vi "Begin.vi"(8 "error in":errorcluster) -> (0 "error out":errorcluster)   [LabVIEW 2020]
doc: "Called before other user functions, this VI is expected to open initial I/O refnums, load in file data, and do all program initialization. Notice that the <B>error out</B> terminal is simply used for data flow. Wiring it to other structures or subVIs ensures that this VI runs first."
uses:
  <vilib>/Rock Robotics/WPI/DriverStation/WPI_DriverStationRobotMode2.ctl
  <vilib>/Rock Robotics/WPI/Joystick/WPI_JoystickDeviceEnum.ctl
  <vilib>/Rock Robotics/WPI/RobotDrive/WPI_RobotDriveDevRef.ctl
  <vilib>/Rock Robotics/WPI/MotorControl/WPI_MotorControlDeviceRef.ctl
  <vilib>/Rock Robotics/WPI/MotorControl/WPI_MotorControlType.ctl
  <vilib>/Rock Robotics/SystemInterfaces/DIO/FPGA_DIOPWMChannel.ctl
  <vilib>/Rock Robotics/WPI/PWM/WPI_PWMDeadband.ctl
  <vilib>/Rock Robotics/SystemInterfaces/DIO/FPGA_DIOChannel.ctl
  <vilib>/Rock Robotics/WPI/SafetyOutput/WPI_SafetyOutputConfigMenu.ctl
  <vilib>/Rock Robotics/WPI/ThirdParty/Phoenix-LabVIEW/Motor Controller/Controls/CTRE_Phoenix_MotorControl_FeedbackDevice.ctl
  <vilib>/Rock Robotics/WPI/ThirdParty/Phoenix-LabVIEW/Motor Controller/Controls/CTRE_Phoenix_MotorControl_NeutralMode.ctl
  <vilib>/Rock Robotics/SystemInterfaces/AI/FPGA_AIChannel.ctl
  <vilib>/Rock Robotics/WPI/ThirdParty/REV Robotics/REVLib/Typedef/Spark MAX Idle Mode.ctl
  Robot Global Data.vi
  <vilib>/Rock Robotics/Network Tables/NT Write String Array.vi
  <vilib>/Rock Robotics/WPI/Switch/WPI_SwitchOpenLimit.vi
  <vilib>/Rock Robotics/WPI/RobotDrive/WPI_RobotDriveOpen2MotorWithTalonSRX.vi
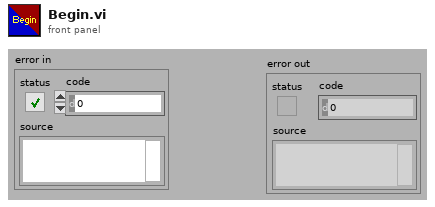
[diagram p1: front panel]
types:
  T1 = typedef "Spark MAX Idle Mode.ctl" = enum16{"Coast", "Brake"}
  T2 = typedef "FPGA_DIOChannel.ctl" = enum8{"DIO 0", "DIO 1", "DIO 2", "DIO 3", "DIO 4", "DIO 5", "DIO 6", "DIO 7", "DIO 8", "DIO 9", "DIO MXP 0", "DIO MXP 1", "DIO MXP 2", "DIO MXP 3", "DIO MXP 4", "DIO MXP 5", "DIO MXP 6", "DIO MXP 7", "DIO MXP 8", "DIO MXP 9", "DIO MXP 10", "DIO MXP 11", "DIO MXP 12", "DIO MXP 13", "DIO MXP 14", "DIO MXP 15", "SPI Port CS1", "SPI Port CS2", "SPI Port CS3", "SPI Port MISO", "SPI Port MOSI", "Invalid"}
  T3 = typedef "FPGA_AIChannel.ctl" = enum8{"AI 0", "AI 1", "AI 2", "AI 3", "AI MXP 0", "AI MXP 1", "AI MXP 2", "AI MXP 3", "Invalid"}
  T4 = typedef "CTRE_Phoenix_MotorControl_FeedbackDevice.ctl" = i8
  T5 = typedef "CTRE_Phoenix_MotorControl_NeutralMode.ctl" = enum8{"EEPROMSetting", "Override to Coast", "Override to Brake"}
  T6 = typedef "WPI_SafetyOutputConfigMenu.ctl" = enum16{"Enable", "Disable"}
  T7 = typedef "WPI_RobotDriveDevRef.ctl" = cluster{"DevStatus":errorcluster, "Motors[]":T8[], "Square Inputs":bool, "Max Output":dbl}
  T8 = typedef "WPI_MotorControlDeviceRef.ctl" = cluster{"DeviceStatus":errorcluster, "Type":T9, "PWM":cluster{"PWM Channel":T10, "DeadBand":T11}, "CAN":cluster{"Device Number":u8, "SetOutput VI Ref":variant, "GetOutput VI Ref":variant, "Enable VI Ref":variant, "Disable VI Ref":variant, "Data":variant}, "Invert":bool, "DIO PWM":cluster{"PWM \"Enable\" Channel":T10, "DIOChannel":T2, "PWM Rate":dbl}}
  T9 = typedef "WPI_MotorControlType.ctl" = enum16{"PWM", "CAN", "DIO PWM"}
  T10 = typedef "FPGA_DIOPWMChannel.ctl" = enum8{"PWM 0", "PWM 1", "PWM 2", "PWM 3", "PWM 4", "PWM 5", "PWM 6", "PWM 7", "PWM 8", "PWM 9", "PWM MXP 0", "PWM MXP 1", "PWM MXP 2", "PWM MXP 3", "PWM MXP 4", "PWM MXP 5", "PWM MXP 6", "PWM MXP 7", "PWM MXP 8", "PWM MXP 9", "Invalid"}
  T11 = typedef "WPI_PWMDeadband.ctl" = cluster{"Name":string, "maxPositivePwm":i32, "minPositivePwm":i32, "centerPwm":i32, "maxNegativePwm":i32, "minNegativePwm":i32, "angularRange":u16}
  T12 = typedef "WPI_JoystickDeviceEnum.ctl" = enum16{"USB 0", "USB 1", "USB 2", "USB 3", "USB 4", "USB 5"}
  T13 = typedef "WPI_DriverStationRobotMode2.ctl" = enum16{"Autonomous Disabled", "Autonomous Enabled", "Teleop Disabled", "Teleop Enabled", "Disconnected", "Finish", "Test Disabled", "Test Enabled", "Emergency Stopped"}
  T14 = typedef "WPI_SwitchDevRef.ctl" = cluster{"DevStatus":errorcluster, "DIO Channel":T2, "CntIndex":T15, "Normally Closed":bool}
  T15 = typedef "FPGA_CounterCtrSystemIndex.ctl" = enum8{"Ctr 0", "Ctr 1", "Ctr 2", "Ctr 3", "Ctr 4", "Ctr 5", "Ctr 6", "Ctr 7", "Invalid"}
  T16 = typedef "WPI_JoystickDevRef.ctl" = cluster{"Device":T12}
  T17 = typedef "WPI_AnalogChannelDevRef.ctl" = cluster{"DevStatus":errorcluster, "Analog Channel":T3}
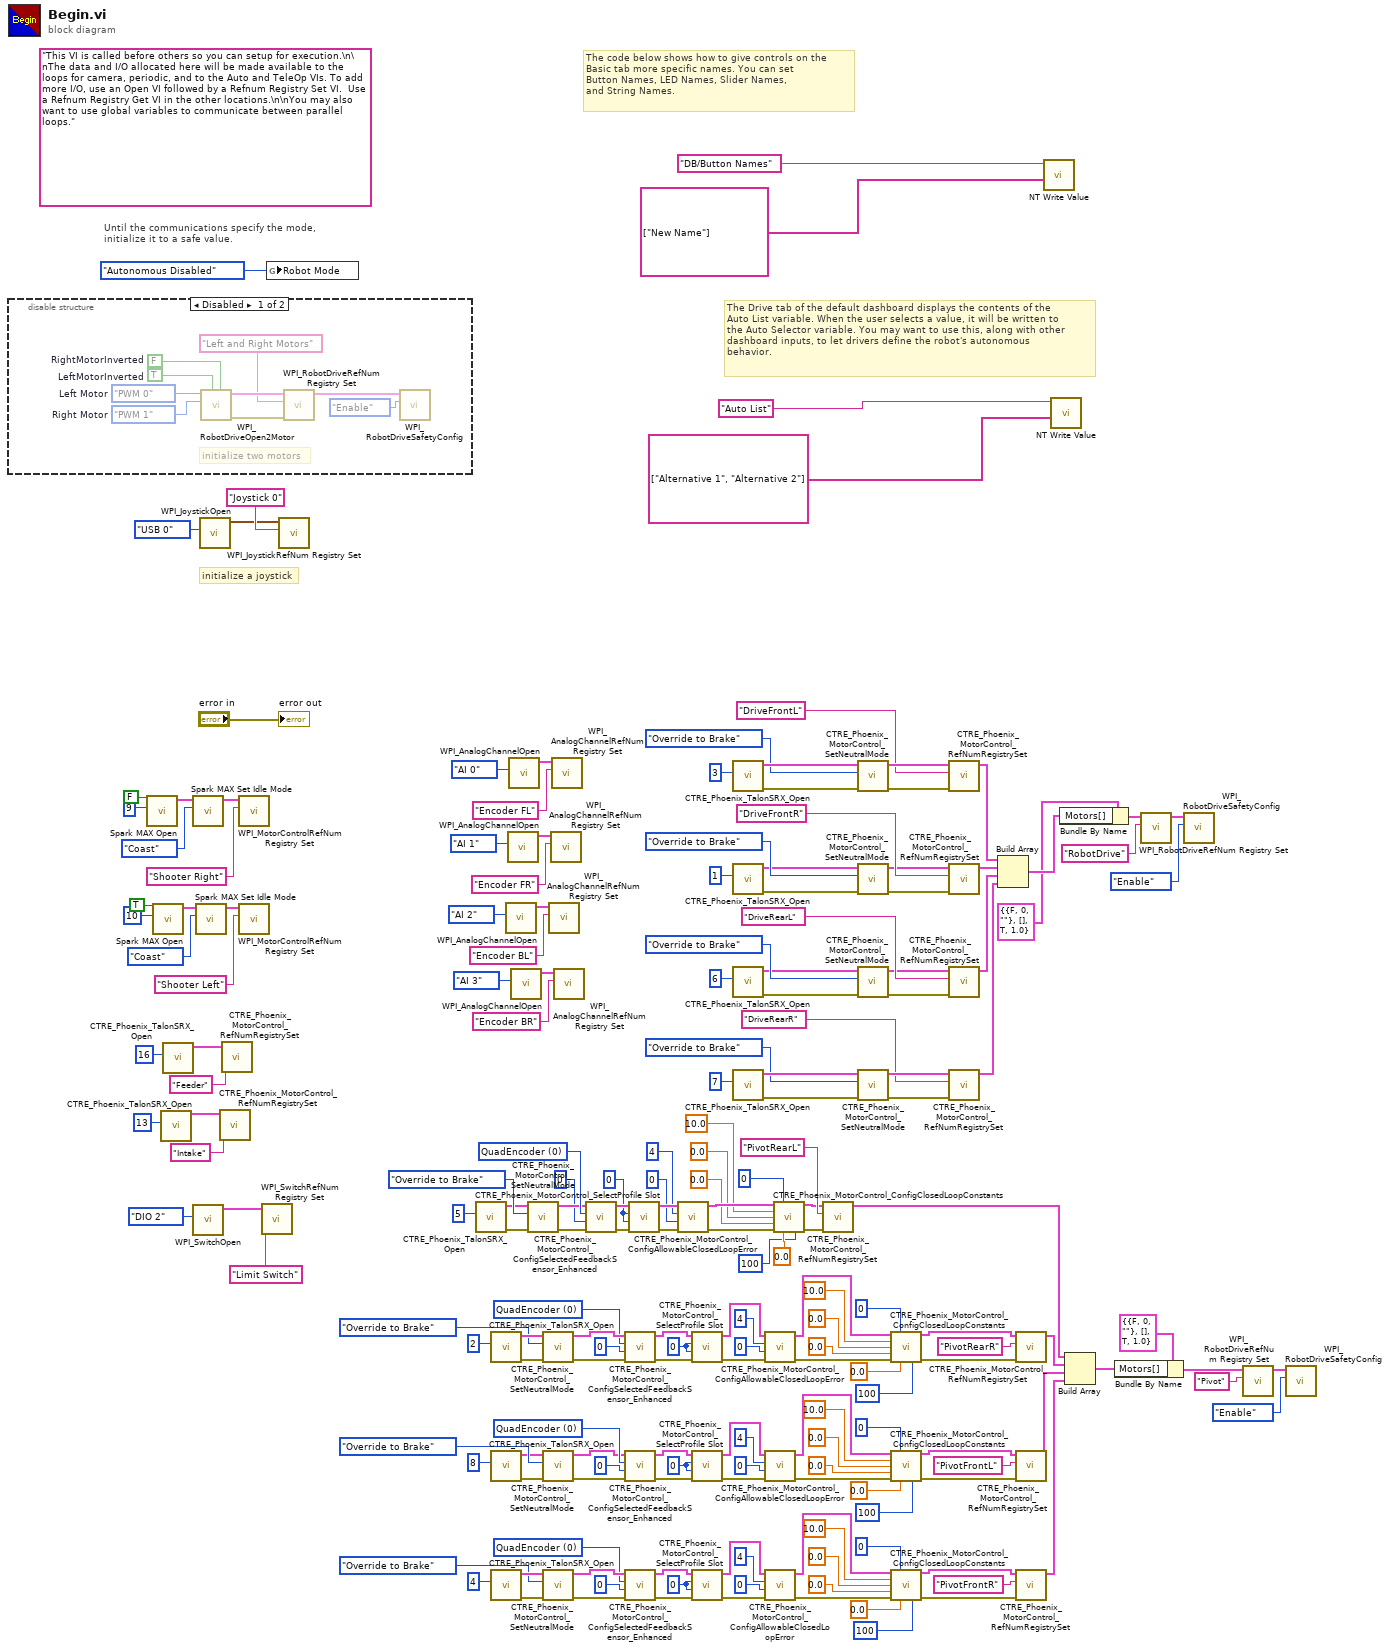
[diagram p0: block diagram]
diagram:
  w50 = 0 ("slotIdx")
  w43 = T4 0 items=["QuadEncoder"=0, "Analog"=2, "Tachometer"=4, "Pulse Width Encoded Position"=8, "Sensor Sum (S0 + S1)"=9, "Sensor Difference (D0 - D1)"=10, "Remote Source 0"=11, "Remote Source 1"=12, "Software Emulated"=15] ("Feedback Device")
  w75 = 0 ("slotIdx")
  w82 = T4 0 items=["QuadEncoder"=0, "Analog"=2, "Tachometer"=4, "Pulse Width Encoded Position"=8, "Sensor Sum (S0 + S1)"=9, "Sensor Difference (D0 - D1)"=10, "Remote Source 0"=11, "Remote Source 1"=12, "Software Emulated"=15] ("Feedback Device")
  w96 = 0 ("slotIdx")
  w89 = T4 0 items=["QuadEncoder"=0, "Analog"=2, "Tachometer"=4, "Pulse Width Encoded Position"=8, "Sensor Sum (S0 + S1)"=9, "Sensor Difference (D0 - D1)"=10, "Remote Source 0"=11, "Remote Source 1"=12, "Software Emulated"=15] ("Feedback Device")
  w123 = 0 ("slotIdx")
  w130 = T4 0 items=["QuadEncoder"=0, "Analog"=2, "Tachometer"=4, "Pulse Width Encoded Position"=8, "Sensor Sum (S0 + S1)"=9, "Sensor Difference (D0 - D1)"=10, "Remote Source 0"=11, "Remote Source 1"=12, "Software Emulated"=15] ("Feedback Device")
  (unwired) "This VI is called before others so you can setup for execution.\n\nThe data and I/O allocated here will be made available to the loops for camera, periodic, and to the Auto and TeleOp VIs. To add more I/O, use an Open VI followed by a Refnum Registry Set VI.  Use a Refnum Registry Get VI in the other locations.\n\nYou may also want to use global variables to communicate between parallel loops."
  # "The Drive tab of the default dashboard displays the contents of the\nAuto List variable. When the user selects a value, it will be written to\nthe Auto Selector variable. You may want to use this, along with other\ndashboard inputs, to let drivers define the robot's autonomous\nbehavior."
  # "The code below shows how to give controls on the\nBasic tab more specific names. You can set\nButton Names, LED Names, Slider Names,\nand String Names."
  # "initialize a joystick"
  # "Until the communications specify the mode,\ninitialize it to a safe value."
  n1 = disable-structure shown="Disabled" {
    frame Disabled {
      w197 = FPGA_DIOPWMChannel."PWM 1"  # Right Motor
      w198 = FPGA_DIOPWMChannel."PWM 0"  # Left Motor
      w202 = TRUE  # LeftMotorInverted
      w203 = FALSE  # RightMotorInverted
      # "initialize two motors"
      n2 = call-poly <vilib>:"WPI_RobotDriveOpen2Motor.vi"("Right Motor Inverted"=w203, "Left Motor Inverted"=w202, "Right Motor"=w197, "Left Motor"=w198) -> ("error out"=w199:errorcluster, "RobotDriveDevRef"=w201:T7)  [unwired: 1 in, 5 out]
      n3 = call <vilib>:"WPI_RobotDriveRefNum Registry Set.vi"("error in (no error)"=w199, "refnum name"="Left and Right Motors", "RobotDriveDevRef"=w201) -> ("RobotDriveDevRef"=w196:T7)  [unwired: 1 in, 7 out]
      n4 = call <vilib>:"WPI_RobotDriveSafetyConfig.vi"("mode"=WPI_SafetyOutputConfigMenu."Enable", "RobotDriveDevRef"=w196) -> ()  [unwired: 8 in, 2 out]
    }
    frame Enabled {
    }
  }
  n5 = call <vilib>:"Spark MAX Open.vi"("Invert"=FALSE, "Device Number"=u8 9) -> ("MotorControlDeviceRef"=w7:T8)  [unwired: 8 in, 1 out]
  n6 = call <vilib>:"Spark MAX Open.vi"("Invert"=TRUE, "Device Number"=u8 10) -> ("MotorControlDeviceRef"=w5:T8)  [unwired: 8 in, 1 out]
  n7 = call <vilib>:"CTRE_Phoenix_TalonSRX_Open.vi"("Device Number"=u8 13) -> ("PhoenixMotorControlDevRef"=w9:T8)  [unwired: 9 in, 1 out]
  n8 = call <vilib>:"CTRE_Phoenix_TalonSRX_Open.vi"("Device Number"=u8 16) -> ("PhoenixMotorControlDevRef"=w16:T8)  [unwired: 9 in, 1 out]
  n9 = call <vilib>:"Spark MAX Set Idle Mode.vi"("Idle Mode"=Spark_MAX_Idle_Mode."Coast", "MotorControlDeviceRef in"=w7) -> ("MotorControlDeviceRef out"=w6:T8)  [unwired: 8 in, 1 out]
  n10 = call-poly <vilib>:"WPI_SwitchOpen.vi"("DIO Channel"=FPGA_DIOChannel."DIO 2") -> ("SwitchDevRef"=w11:T14)  [unwired: 9 in, 1 out]
  n11 = call <vilib>:"Spark MAX Set Idle Mode.vi"("Idle Mode"=Spark_MAX_Idle_Mode."Coast", "MotorControlDeviceRef in"=w5) -> ("MotorControlDeviceRef out"=w3:T8)  [unwired: 8 in, 1 out]
  n12 = call <vilib>:"WPI_JoystickOpen.vi"("JoystickDevice"=WPI_JoystickDeviceEnum."USB 0") -> ("JoystickDevRef"=w192:T16)  [unwired: 10 in]
  n13 = call <vilib>:"CTRE_Phoenix_MotorControl_RefNumRegistrySet.vi"("refnum name"="Intake", "PhoenixMotorControlDevRef"=w9) -> ()  [unwired: 8 in, 2 out]
  n14 = call <vilib>:"CTRE_Phoenix_MotorControl_RefNumRegistrySet.vi"("refnum name"="Feeder", "PhoenixMotorControlDevRef"=w16) -> ()  [unwired: 8 in, 2 out]
  n15 = call <vilib>:"WPI_MotorControlRefNum Registry Set.vi"("refnum name"="Shooter Right", "MotorControlDevRef"=w6) -> ()  [unwired: 8 in, 2 out]
  n16 = call <vilib>:"WPI_MotorControlRefNum Registry Set.vi"("refnum name"="Shooter Left", "MotorControlDevRef"=w3) -> ()  [unwired: 8 in, 2 out]
  n17 = call <vilib>:"WPI_SwitchRefNum Registry Set.vi"("refnum name"="Limit Switch", "SwitchDevRef"=w11) -> ()  [unwired: 8 in, 2 out]
  n18 = global write "Robot Global Data.vi" "Robot Mode"(WPI_DriverStationRobotMode2."Autonomous Disabled" ("Robot Mode")) -> ()
  n19 = call <vilib>:"WPI_JoystickRefNum Registry Set.vi"("refnum name"="Joystick 0", "JoystickDevRef"=w192) -> ()  [unwired: 8 in, 2 out]
  n20 = call <vilib>:"CTRE_Phoenix_TalonSRX_Open.vi"("Device Number"=5) -> ("error out"=w127:errorcluster, "PhoenixMotorControlDevRef"=w164:T8)  [unwired: 9 in]
  n21 = call <vilib>:"CTRE_Phoenix_TalonSRX_Open.vi"("Device Number"=2) -> ("error out"=w92:errorcluster, "PhoenixMotorControlDevRef"=w87:T8)  [unwired: 9 in]
  n22 = call <vilib>:"CTRE_Phoenix_TalonSRX_Open.vi"("Device Number"=8) -> ("error out"=w79:errorcluster, "PhoenixMotorControlDevRef"=w84:T8)  [unwired: 9 in]
  n23 = call <vilib>:"CTRE_Phoenix_TalonSRX_Open.vi"("Device Number"=4) -> ("error out"=w46:errorcluster, "PhoenixMotorControlDevRef"=w41:T8)  [unwired: 9 in]
  n24 = call <vilib>:"WPI_AnalogChannelOpen.vi"("Analog Channel"=FPGA_AIChannel."AI 2") -> ("AIDeviceRef"=w28:T17)  [unwired: 9 in, 1 out]
  n25 = call <vilib>:"WPI_AnalogChannelOpen.vi"("Analog Channel"=FPGA_AIChannel."AI 1") -> ("AIDeviceRef"=w25:T17)  [unwired: 9 in, 1 out]
  n26 = call <vilib>:"WPI_AnalogChannelOpen.vi"("Analog Channel"=FPGA_AIChannel."AI 0") -> ("AIDeviceRef"=w23:T17)  [unwired: 9 in, 1 out]
  n27 = call <vilib>:"WPI_AnalogChannelOpen.vi"("Analog Channel"=FPGA_AIChannel."AI 3") -> ("AIDeviceRef"=w29:T17)  [unwired: 9 in, 1 out]
  n28 = call <vilib>:"CTRE_Phoenix_MotorControl_SetNeutralMode.vi"("error in (no error)"=w127, "Motor Control Neutral Mode"=CTRE_Phoenix_MotorControl_NeutralMode."Override to Brake", "PhoenixMotorControlDevRef"=w164) -> ("error out"=w126:errorcluster, "PhoenixMotorControlDevRef"=w129:T8)  [unwired: 7 in]
  n29 = call <vilib>:"CTRE_Phoenix_MotorControl_SetNeutralMode.vi"("error in (no error)"=w92, "Motor Control Neutral Mode"=CTRE_Phoenix_MotorControl_NeutralMode."Override to Brake", "PhoenixMotorControlDevRef"=w87) -> ("error out"=w93:errorcluster, "PhoenixMotorControlDevRef"=w90:T8)  [unwired: 7 in]
  n30 = call <vilib>:"CTRE_Phoenix_MotorControl_SetNeutralMode.vi"("error in (no error)"=w79, "Motor Control Neutral Mode"=CTRE_Phoenix_MotorControl_NeutralMode."Override to Brake", "PhoenixMotorControlDevRef"=w84) -> ("error out"=w78:errorcluster, "PhoenixMotorControlDevRef"=w81:T8)  [unwired: 7 in]
  n31 = call <vilib>:"CTRE_Phoenix_MotorControl_SetNeutralMode.vi"("error in (no error)"=w46, "Motor Control Neutral Mode"=CTRE_Phoenix_MotorControl_NeutralMode."Override to Brake", "PhoenixMotorControlDevRef"=w41) -> ("error out"=w47:errorcluster, "PhoenixMotorControlDevRef"=w44:T8)  [unwired: 7 in]
  n32 = call <vilib>:"WPI_AnalogChannelRefNum Registry Set.vi"("refnum name"="Encoder BL", "AIDeviceRef"=w28) -> ()  [unwired: 8 in, 2 out]
  n33 = call <vilib>:"WPI_AnalogChannelRefNum Registry Set.vi"("refnum name"="Encoder FR", "AIDeviceRef"=w25) -> ()  [unwired: 8 in, 2 out]
  n34 = call <vilib>:"WPI_AnalogChannelRefNum Registry Set.vi"("refnum name"="Encoder FL", "AIDeviceRef"=w23) -> ()  [unwired: 8 in, 2 out]
  n35 = call <vilib>:"WPI_AnalogChannelRefNum Registry Set.vi"("refnum name"="Encoder BR", "AIDeviceRef"=w29) -> ()  [unwired: 8 in, 2 out]
  n36 = call <vilib>:"CTRE_Phoenix_MotorControl_ConfigSelectedFeedbackSensor_Enhanced.vi"("error in (no error)"=w126, "pidLoopIdx"=0, "Feedback Device"=w130, "PhoenixMotorControlDevRef"=w129) -> ("error out"=w125:errorcluster, "PhoenixMotorControlDevRef"=w124:T8)  [unwired: 6 in]
  n37 = call <vilib>:"CTRE_Phoenix_MotorControl_ConfigSelectedFeedbackSensor_Enhanced.vi"("error in (no error)"=w93, "pidLoopIdx"=0, "Feedback Device"=w89, "PhoenixMotorControlDevRef"=w90) -> ("error out"=w94:errorcluster, "PhoenixMotorControlDevRef"=w95:T8)  [unwired: 6 in]
  n38 = call <vilib>:"CTRE_Phoenix_MotorControl_ConfigSelectedFeedbackSensor_Enhanced.vi"("error in (no error)"=w78, "pidLoopIdx"=0, "Feedback Device"=w82, "PhoenixMotorControlDevRef"=w81) -> ("error out"=w77:errorcluster, "PhoenixMotorControlDevRef"=w76:T8)  [unwired: 6 in]
  n39 = call <vilib>:"CTRE_Phoenix_MotorControl_ConfigSelectedFeedbackSensor_Enhanced.vi"("error in (no error)"=w47, "pidLoopIdx"=0, "Feedback Device"=w43, "PhoenixMotorControlDevRef"=w44) -> ("error out"=w48:errorcluster, "PhoenixMotorControlDevRef"=w49:T8)  [unwired: 6 in]
  n40 = call <vilib>:"CTRE_Phoenix_MotorControl_SelectProfile Slot.vi"("error in (no error)"=w125, "pidLoopIdx"=w123, "slotIdx"=w123, "PhoenixMotorControlDevRef"=w124) -> ("error out"=w122:errorcluster, "PhoenixMotorControlDevRef"=w121:T8)  [unwired: 6 in]
  n41 = call <vilib>:"CTRE_Phoenix_MotorControl_ConfigAllowableClosedLoopError.vi"("error in (no error)"=w122, "slotIdx"=u32 0, "allowableClosedLoopError"=4, "PhoenixMotorControlDevRef"=w121) -> ("error out"=w117:errorcluster, "PhoenixMotorControlDevRef"=w118:T8)  [unwired: 6 in]
  n42 = call <vilib>:"CTRE_Phoenix_MotorControl_SelectProfile Slot.vi"("error in (no error)"=w94, "pidLoopIdx"=w96, "slotIdx"=w96, "PhoenixMotorControlDevRef"=w95) -> ("error out"=w97:errorcluster, "PhoenixMotorControlDevRef"=w98:T8)  [unwired: 6 in]
  n43 = call <vilib>:"CTRE_Phoenix_MotorControl_SelectProfile Slot.vi"("error in (no error)"=w77, "pidLoopIdx"=w75, "slotIdx"=w75, "PhoenixMotorControlDevRef"=w76) -> ("error out"=w74:errorcluster, "PhoenixMotorControlDevRef"=w73:T8)  [unwired: 6 in]
  n44 = call <vilib>:"CTRE_Phoenix_MotorControl_SelectProfile Slot.vi"("error in (no error)"=w48, "pidLoopIdx"=w50, "slotIdx"=w50, "PhoenixMotorControlDevRef"=w49) -> ("error out"=w51:errorcluster, "PhoenixMotorControlDevRef"=w52:T8)  [unwired: 6 in]
  n45 = call <vilib>:"CTRE_Phoenix_TalonSRX_Open.vi"("Device Number"=3) -> ("error out"=w182:errorcluster, "PhoenixMotorControlDevRef"=w181:T8)  [unwired: 9 in]
  n46 = call <vilib>:"CTRE_Phoenix_TalonSRX_Open.vi"("Device Number"=1) -> ("error out"=w157:errorcluster, "PhoenixMotorControlDevRef"=w158:T8)  [unwired: 9 in]
  n47 = call <vilib>:"CTRE_Phoenix_TalonSRX_Open.vi"("Device Number"=6) -> ("error out"=w143:errorcluster, "PhoenixMotorControlDevRef"=w144:T8)  [unwired: 9 in]
  n48 = call <vilib>:"CTRE_Phoenix_TalonSRX_Open.vi"("Device Number"=7) -> ("error out"=w150:errorcluster, "PhoenixMotorControlDevRef"=w149:T8)  [unwired: 9 in]
  n49 = call <vilib>:"CTRE_Phoenix_MotorControl_ConfigAllowableClosedLoopError.vi"("error in (no error)"=w97, "slotIdx"=u32 0, "allowableClosedLoopError"=4, "PhoenixMotorControlDevRef"=w98) -> ("error out"=w102:errorcluster, "PhoenixMotorControlDevRef"=w101:T8)  [unwired: 6 in]
  n50 = call <vilib>:"CTRE_Phoenix_MotorControl_ConfigAllowableClosedLoopError.vi"("error in (no error)"=w74, "slotIdx"=u32 0, "allowableClosedLoopError"=4, "PhoenixMotorControlDevRef"=w73) -> ("error out"=w69:errorcluster, "PhoenixMotorControlDevRef"=w70:T8)  [unwired: 6 in]
  n51 = call <vilib>:"CTRE_Phoenix_MotorControl_ConfigAllowableClosedLoopError.vi"("error in (no error)"=w51, "slotIdx"=u32 0, "allowableClosedLoopError"=4, "PhoenixMotorControlDevRef"=w52) -> ("error out"=w56:errorcluster, "PhoenixMotorControlDevRef"=w55:T8)  [unwired: 6 in]
  n52 = call <vilib>:"CTRE_Phoenix_MotorControl_ConfigClosedLoopConstants.vi"("PhoenixMotorControlDevRef"=w118, "slotIdx"=0, "P"=10.0, "I"=0.0, "D"=0.0, "error in (no error)"=w117, "F"=0.0, "timeoutMs"=100) -> ("PhoenixMotorControlDevRef"=w110:T8, "error out"=w109:errorcluster)  [unwired: 6 in]
  n53 = call <vilib>:"CTRE_Phoenix_MotorControl_RefNumRegistrySet.vi"("error in (no error)"=w109, "refnum name"="PivotRearL", "PhoenixMotorControlDevRef"=w110) -> ("PhoenixMotorControlDevRef"=w170:T8)  [unwired: 7 in, 1 out]
  n54 = call <vilib>:"CTRE_Phoenix_MotorControl_SetNeutralMode.vi"("error in (no error)"=w182, "Motor Control Neutral Mode"=CTRE_Phoenix_MotorControl_NeutralMode."Override to Brake", "PhoenixMotorControlDevRef"=w181) -> ("error out"=w184:errorcluster, "PhoenixMotorControlDevRef"=w183:T8)  [unwired: 7 in]
  n55 = call <vilib>:"CTRE_Phoenix_MotorControl_SetNeutralMode.vi"("error in (no error)"=w157, "Motor Control Neutral Mode"=CTRE_Phoenix_MotorControl_NeutralMode."Override to Brake", "PhoenixMotorControlDevRef"=w158) -> ("error out"=w155:errorcluster, "PhoenixMotorControlDevRef"=w156:T8)  [unwired: 7 in]
  n56 = call <vilib>:"CTRE_Phoenix_MotorControl_SetNeutralMode.vi"("error in (no error)"=w143, "Motor Control Neutral Mode"=CTRE_Phoenix_MotorControl_NeutralMode."Override to Brake", "PhoenixMotorControlDevRef"=w144) -> ("error out"=w141:errorcluster, "PhoenixMotorControlDevRef"=w142:T8)  [unwired: 7 in]
  n57 = call <vilib>:"CTRE_Phoenix_MotorControl_SetNeutralMode.vi"("error in (no error)"=w150, "Motor Control Neutral Mode"=CTRE_Phoenix_MotorControl_NeutralMode."Override to Brake", "PhoenixMotorControlDevRef"=w149) -> ("error out"=w152:errorcluster, "PhoenixMotorControlDevRef"=w151:T8)  [unwired: 7 in]
  n58 = call <vilib>:"CTRE_Phoenix_MotorControl_ConfigClosedLoopConstants.vi"("PhoenixMotorControlDevRef"=w101, "slotIdx"=0, "P"=10.0, "I"=0.0, "D"=0.0, "error in (no error)"=w102, "F"=0.0, "timeoutMs"=100) -> ("PhoenixMotorControlDevRef"=w34:T8, "error out"=w35:errorcluster)  [unwired: 6 in]
  n59 = call <vilib>:"CTRE_Phoenix_MotorControl_ConfigClosedLoopConstants.vi"("PhoenixMotorControlDevRef"=w70, "slotIdx"=0, "P"=10.0, "I"=0.0, "D"=0.0, "error in (no error)"=w69, "F"=0.0, "timeoutMs"=100) -> ("PhoenixMotorControlDevRef"=w37:T8, "error out"=w36:errorcluster)  [unwired: 6 in]
  n60 = call <vilib>:"CTRE_Phoenix_MotorControl_ConfigClosedLoopConstants.vi"("PhoenixMotorControlDevRef"=w55, "slotIdx"=0, "P"=10.0, "I"=0.0, "D"=0.0, "error in (no error)"=w56, "F"=0.0, "timeoutMs"=100) -> ("PhoenixMotorControlDevRef"=w39:T8, "error out"=w38:errorcluster)  [unwired: 6 in]
  n61 = call <vilib>:"CTRE_Phoenix_MotorControl_RefNumRegistrySet.vi"("error in (no error)"=w184, "refnum name"="DriveFrontL", "PhoenixMotorControlDevRef"=w183) -> ("PhoenixMotorControlDevRef"=w177:T8)  [unwired: 7 in, 1 out]
  n62 = call <vilib>:"CTRE_Phoenix_MotorControl_RefNumRegistrySet.vi"("error in (no error)"=w155, "refnum name"="DriveFrontR", "PhoenixMotorControlDevRef"=w156) -> ("PhoenixMotorControlDevRef"=w136:T8)  [unwired: 7 in, 1 out]
  n63 = call <vilib>:"CTRE_Phoenix_MotorControl_RefNumRegistrySet.vi"("error in (no error)"=w141, "refnum name"="DriveRearL", "PhoenixMotorControlDevRef"=w142) -> ("PhoenixMotorControlDevRef"=w135:T8)  [unwired: 7 in, 1 out]
  n64 = call <vilib>:"CTRE_Phoenix_MotorControl_RefNumRegistrySet.vi"("error in (no error)"=w152, "refnum name"="DriveRearR", "PhoenixMotorControlDevRef"=w151) -> ("PhoenixMotorControlDevRef"=w134:T8)  [unwired: 7 in, 1 out]
  n65 = Build Array(w177, w136, w135, w134) -> (w176:T8[])
  n66 = call <vilib>:"CTRE_Phoenix_MotorControl_RefNumRegistrySet.vi"("error in (no error)"=w35, "refnum name"="PivotRearR", "PhoenixMotorControlDevRef"=w34) -> ("PhoenixMotorControlDevRef"=w133:T8)  [unwired: 7 in, 1 out]
  n67 = call <vilib>:"CTRE_Phoenix_MotorControl_RefNumRegistrySet.vi"("error in (no error)"=w36, "refnum name"="PivotFrontL", "PhoenixMotorControlDevRef"=w37) -> ("PhoenixMotorControlDevRef"=w132:T8)  [unwired: 7 in, 1 out]
  n68 = call <vilib>:"CTRE_Phoenix_MotorControl_RefNumRegistrySet.vi"("error in (no error)"=w38, "refnum name"="PivotFrontR", "PhoenixMotorControlDevRef"=w39) -> ("PhoenixMotorControlDevRef"=w131:T8)  [unwired: 7 in, 1 out]
  n69 = call-poly <vilib>:"NT Write Value.vi"("String Array"=string[] ["New Name"], "Name"="DB/Button Names") -> ()  [unwired: 9 in, 1 out]
  n70 = call-poly <vilib>:"NT Write Value.vi"("String Array"=string[] ["Alternative 1", "Alternative 2"], "Name"="Auto List") -> ()  [unwired: 9 in, 1 out]
  n71 = Bundle By Name(cluster=T7 {"DevStatus"={"status"=FALSE, "code"=0, "source"=""}, "Motors[]"=[], "Square Inputs"=TRUE, "Max Output"=1.0} ("RobotDriveDevRef"), "Motors[]"=w176) -> (w161:T7)
  n72 = Build Array(w170, w133, w132, w131) -> (w171:T8[])
  n73 = Bundle By Name(cluster=T7 {"DevStatus"={"status"=FALSE, "code"=0, "source"=""}, "Motors[]"=[], "Square Inputs"=TRUE, "Max Output"=1.0} ("RobotDriveDevRef"), "Motors[]"=w171) -> (w168:T7)
  n74 = call <vilib>:"WPI_RobotDriveRefNum Registry Set.vi"("refnum name"="RobotDrive", "RobotDriveDevRef"=w161) -> ("RobotDriveDevRef"=w175:T7)  [unwired: 8 in, 1 out]
  n75 = call <vilib>:"WPI_RobotDriveSafetyConfig.vi"("mode"=WPI_SafetyOutputConfigMenu."Enable", "RobotDriveDevRef"=w175) -> ()  [unwired: 8 in, 2 out]
  n76 = call <vilib>:"WPI_RobotDriveRefNum Registry Set.vi"("refnum name"="Pivot", "RobotDriveDevRef"=w168) -> ("RobotDriveDevRef"=w172:T7)  [unwired: 8 in, 1 out]
  n77 = call <vilib>:"WPI_RobotDriveSafetyConfig.vi"("mode"=WPI_SafetyOutputConfigMenu."Enable", "RobotDriveDevRef"=w172) -> ()  [unwired: 8 in, 2 out]
  "error out" <- "error in"
